vi "Drivetrain Loop.vi"   [LabVIEW 2014]
uses:
  Common Code/Drivetrain Status.ctl
  Drivetrain Mode.ctl
  Common Code/Dist Drive Status.ctl
  Common Code/Change Detect Int.vi
  Common Code/Change Detect Boolean.vi
  Robot Global Data.vi
types:
  T1 = typedef "Drivetrain Status.ctl" = cluster{"Y (Throttle)":sgl, "X (Steer)":sgl, "Translation X":sgl, "Center Wheel Down":bool, "Mode":T2, "Distance Drive finished?":bool, "Y Target":sgl, "X Target":sgl, "Heading Target":sgl, "Dist Drive Status":T3}
  T2 = typedef "Drivetrain Mode.ctl" = enum16{"Manual", "Gyro Steer", "Vision Steer", "Drive Distance"}
  T3 = typedef "Dist Drive Status.ctl" = cluster{"Y In Range":bool, "X In Range":bool, "Gyro In Range":bool, "Y Dist":dbl, "X Dist":dbl, "Gyro":dbl}
  T4 = typedef "Drivetrain Control.ctl" = cluster{"Mode":T2, "Steer":dbl, "Y":dbl, "Heading Target":dbl, "Strafe X":dbl, "Y Target":dbl, "Strafe Target":dbl}
  T5 = typedef "WPI_DriverStationRobotMode2.ctl" = enum16{"Autonomous Disabled", "Autonomous Enabled", "Teleop Disabled", "Teleop Enabled", "Disconnected", "Finish", "Test Disabled", "Test Enabled", "Emergency Stopped"}
  T6 = typedef "WPI_MotorControlDeviceRef.ctl" = cluster{"DeviceStatus":errorcluster, "Type":T7, "PWM":cluster{"Controller":T8, "PWM Channel":T9, "DeadBand":T10}, "CAN":cluster{"Device Number":u8, "Control Mode":T11, "Semaphore":T12, "Max Vout":dbl, "TalonSRX Control Mode":T13}, "Invert":bool, "TransformRef":T14, "InvTransformRef":T14}
  T7 = typedef "WPI_MotorControlType.ctl" = enum16{"PWM", "CAN", "CANTalonSRX"}
  T8 = typedef "FPGA_TypedefDigitalModule.ctl" = enum16{"Controller 1"}
  T9 = typedef "FPGA_DIOPWMChannel.ctl" = enum8{"PWM 0", "PWM 1", "PWM 2", "PWM 3", "PWM 4", "PWM 5", "PWM 6", "PWM 7", "PWM 8", "PWM 9", "PWM MXP 0", "PWM MXP 1", "PWM MXP 2", "PWM MXP 3", "PWM MXP 4", "PWM MXP 5", "PWM MXP 6", "PWM MXP 7", "PWM MXP 8", "PWM MXP 9", "Invalid"}
  T10 = typedef "WPI_PWMDeadband.ctl" = cluster{"Name":string, "maxPositivePwm":i32, "minPositivePwm":i32, "centerPwm":i32, "maxNegativePwm":i32, "minNegativePwm":i32, "angularRange":u16}
  T11 = typedef "WPI_CANJaguar_ControlMode.ctl" = enum8{"Percent VBus", "Current", "Speed", "Position", "Voltage"}
  T12 = typedef "Semaphore RefNum" = refnum<k1>
  T13 = typedef "WPI_CANTalonSRX_APIControlMode.ctl" = enum8{"Percent VBus", "Speed", "Position", "Slave", "Unchanged / Invalid"}
  T14 = typedef "WPI_PWMTransform_ConPane.ctl" = refnum<vi>
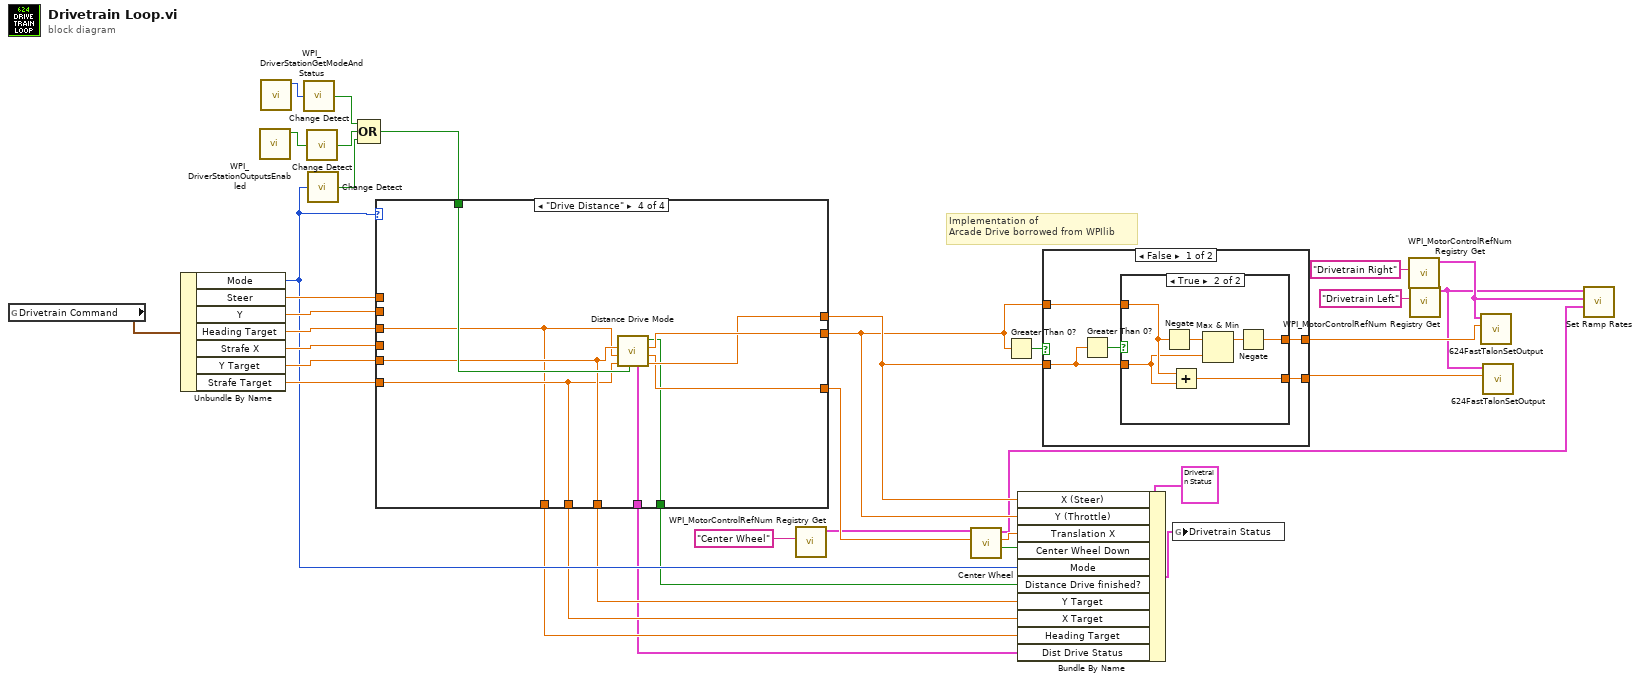
[diagram p0: block diagram]
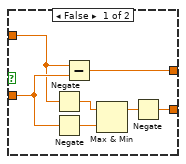
[diagram p2: hidden frame]
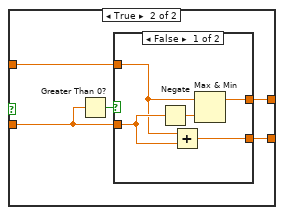
[diagram p3: hidden frame]
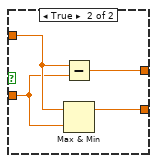
[diagram p4: hidden frame]
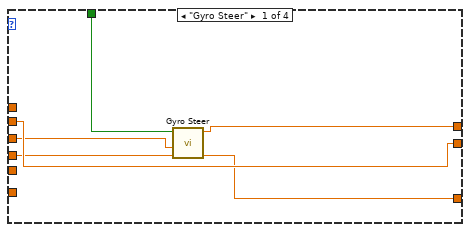
[diagram p5: hidden frame]
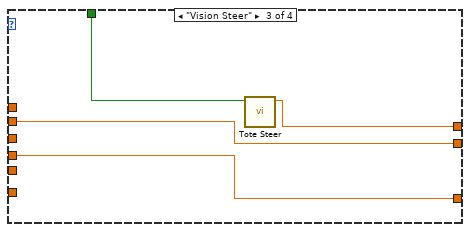
[diagram p7: hidden frame]
diagram:
  # "Implementation of \nArcade Drive borrowed from WPIlib"
  n1 = global read "Robot Global Data.vi" "Drivetrain Command"() -> (w34:T4)
  n2 = Unbundle By Name(w34) -> ("Mode"=w22:T2, "Steer"=w33:dbl, "Y"=w36:dbl, "Heading Target"=w35:dbl, "Strafe X"=w32:dbl, "Y Target"=w31:dbl, "Strafe Target"=w30:dbl)
  n3 = call <vilib>:"WPI_DriverStationOutputsEnabled.vi"() -> ("OutputsEnabled?"=w20:bool)  [unwired: 10 in, 1 out]
  n4 = call <vilib>:"WPI_DriverStationGetModeAndStatus.vi"() -> ("Robot Mode"=w21:T5)  [unwired: 10 in, 1 out]
  n5 = call-poly "Change Detect.vi"("In"=w21) -> ("Changed?"=w17:bool)
  n6 = call-poly "Change Detect.vi"("In"=w20) -> ("Changed?"=w18:bool)
  n7 = call-poly "Change Detect.vi"("In"=w22) -> ("Changed?"=w19:bool)
  n8 = Compound Arithmetic op=OR(w17, w18, w19) -> (w16:bool)
  n9 = case shown="\"Drive Distance\"" w22 {
    tunnel: [w40 w44 w48 w56] -> w26
    tunnel: w33 -> [_ w44 _ _]
    tunnel: [w41 w43 w47 w57] -> w25
    tunnel: w36 -> [w41 w43 w47 _]
    tunnel: w35 -> [w39 _ _ w50]
    tunnel: w32 -> [w38 w42 w46 _]
    tunnel: [w38 w42 w46 w55] -> w29
    tunnel: w31 -> [_ _ _ w52]
    tunnel: w30 -> [_ _ _ w51]
    tunnel: w16 -> [w37 _ w45 w54]
    tunnel: [_ _ _ w53] -> w15
    tunnel: [_ _ _ w52] -> w14
    tunnel: [_ _ _ w51] -> w13
    tunnel: [_ _ _ w50] -> w12
    tunnel: [_ _ _ w49] -> w11
    frame "Gyro Steer" {
      n10 = call "Gyro Steer.vi"("Target Angle"=w39, "Changed?"=w37) -> ("X out"=w40:dbl)  [unwired: 8 in, 1 out]
    }
    frame "Manual", Default {
    }
    frame "Vision Steer" {
      n11 = call "Tote Steer.vi"("Changed?"=w45) -> ("f"=w48:dbl)  [unwired: 10 in]
    }
    frame "Drive Distance" {
      n12 = call "Distance Drive Mode.vi"("Reinitialize"=w54, "Strafe target"=w51, "Heading target"=w50, "Y target"=w52) -> ("X out"=w56:dbl, "Strafe out"=w55:dbl, "Y out"=w57:dbl, "isFinished"=w53:bool, "Dist Drive Status"=w49:T3)  [unwired: 3 in]
    }
  }
  n13 = call <vilib>:"WPI_MotorControlRefNum Registry Get.vi"("refnum name"="Center Wheel") -> ("MotorControlDevRef"=w4:T6)  [unwired: 9 in, 1 out]
  n14 = call "Center Wheel.vi"("Center Wheel Value"=w29, "MotorControlDevRef"=w4) -> ("Wheel Down"=w23:bool, "X Out"=w24:dbl, "MotorControlDevRef 2"=w3:T6)  [unwired: 7 in]
  n15 = Greater Than 0?(x=w25) -> (x > 0?=w10:bool)
  n16 = Bundle By Name(cluster=T1 {"Y (Throttle)"=0.0, "X (Steer)"=0.0, "Translation X"=0.0, "Center Wheel Down"=FALSE, "Mode"=enum."Manual", "Distance Drive finished?"=FALSE, "Y Target"=0.0, "X Target"=0.0, "Heading Target"=0.0, "Dist Drive Status"={"Y In Range"=FALSE, "X In Range"=FALSE, "Gyro In Range"=FALSE, "Y Dist"=0.0, "X Dist"=0.0, "Gyro"=0.0}} ("Drivetrain Status"), "X (Steer)"=w26, "Y (Throttle)"=w25, "Translation X"=w24, "Center Wheel Down"=w23, "Mode"=w22, "Distance Drive finished?"=w15, "Y Target"=w14, "X Target"=w13, "Heading Target"=w12, "Dist Drive Status"=w11) -> (w28:T1)
  n17 = case shown="False" w10 {
    tunnel: w26 -> [w61 w79]
    tunnel: w25 -> [w60 w78]
    tunnel: [w59 w77] -> w7
    tunnel: [w58 w76] -> w6
    frame False {
      n18 = Greater Than 0?(x=w61) -> (x > 0?=w62:bool)
      n19 = case shown="True" w62 {
        tunnel: w61 -> [w69 w71]
        tunnel: w60 -> [w67 w72]
        tunnel: [w63 w73] -> w59
        tunnel: [w64 w70] -> w58
        frame False {
          n20 = Negate(x=w67) -> (-x=w68:dbl)
          n21 = Negate(x=w69) -> (-x=w66:dbl)
          n22 = Subtract(x=w67, y=w69) -> (x-y=w63:dbl)
          n23 = Max & Min(x=w68, y=w66) -> (max(x,y)=w65:dbl)  [unwired: 1 out]
          n24 = Negate(x=w65) -> (-x=w64:dbl)
        }
        frame True {
          n25 = Negate(x=w72) -> (-x=w75:dbl)
          n26 = Add(x=w72, y=w71) -> (x+y=w70:dbl)
          n27 = Max & Min(x=w75, y=w71) -> (max(x,y)=w74:dbl)  [unwired: 1 out]
          n28 = Negate(x=w74) -> (-x=w73:dbl)
        }
      }
    }
    frame True {
      n29 = Greater Than 0?(x=w79) -> (x > 0?=w80:bool)
      n30 = case shown="False" w80 {
        tunnel: w79 -> [w85 w87]
        tunnel: w78 -> [w82 w88]
        tunnel: [w83 w86] -> w77
        tunnel: [w81 w89] -> w76
        frame False {
          n31 = Negate(x=w85) -> (-x=w84:dbl)
          n32 = Add(x=w82, y=w85) -> (x+y=w81:dbl)
          n33 = Max & Min(x=w82, y=w84) -> (max(x,y)=w83:dbl)  [unwired: 1 out]
        }
        frame True {
          n34 = Subtract(x=w88, y=w87) -> (x-y=w86:dbl)
          n35 = Max & Min(x=w88, y=w87) -> (max(x,y)=w89:dbl)  [unwired: 1 out]
        }
      }
    }
  }
  n36 = global write "Robot Global Data.vi" "Drivetrain Status"(w28) -> ()
  n37 = call <vilib>:"WPI_MotorControlRefNum Registry Get.vi"("refnum name"="Drivetrain Right") -> ("MotorControlDevRef"=w2:T6)  [unwired: 9 in, 1 out]
  n38 = call <vilib>:"WPI_MotorControlRefNum Registry Get.vi"("refnum name"="Drivetrain Left") -> ("MotorControlDevRef"=w1:T6)  [unwired: 9 in, 1 out]
  n39 = call "624FastTalonSetOutput.vi"("Output"=w7, "MotorControlDevRef"=w2) -> ()  [unwired: 8 in, 2 out]
  n40 = call "624FastTalonSetOutput.vi"("Output"=w6, "MotorControlDevRef"=w1) -> ()  [unwired: 8 in, 2 out]
  n41 = call "Set Ramp Rates.vi"("DT Center"=w3, "DT Right"=w2, "DT Left"=w1) -> ()  [unwired: 9 in]
